vi "Create Custom Device.vi"(0 "Name":string, 5 "AIT 1553 Settings":T2={"Board Serial #"=685, "AppLicense"=FALSE, "License Key"="", "BusEnabledProperties"={"Bus1Enabled"=TRUE, "Bus2Enabled"=FALSE, "Bus3Enabled"=FALSE, "Bus4Enabled"=FALSE}, "Description"="Driver for AIT 1553 Device for VeriStand", "Bus1 Path"=path "", "Bus2 Path"=path "", "Bus3 Path"=path "", "Bus4 Path"=path ""}, 11 "error in (no error)":errorcluster) -> (4 "Custom Device reference":refnum<k24>, 15 "error out":errorcluster)   [LabVIEW 2011]
uses:
  NationalInstruments.VeriStand.SystemDefinitionAPI
  Controls/AIT 1553 Settings.ctl
  System Explorer/Controls/1553 Bus Enabled.ctl
  <vilib>/NI Veristand/Custom Device API/Custom Device Item Ref.ctl
  Controls and Global/Global.vi
  <vilib>/NI Veristand/Custom Device API/Set Item Property (Boolean).vi
  <vilib>/NI Veristand/Custom Device API/Set Item Property (String).vi
  <vilib>/NI Veristand/Custom Device API/Set Item Property (Variant).vi
  <vilib>/NI Veristand/Custom Device API/Custom Device API.lvlib
  AIT 1553 Custom Device.lvlib
panel:
  out "Sim Filenames":path[](array[path])
  out "Bus Nodes":T1[](array[typedef]) format="%.0x"
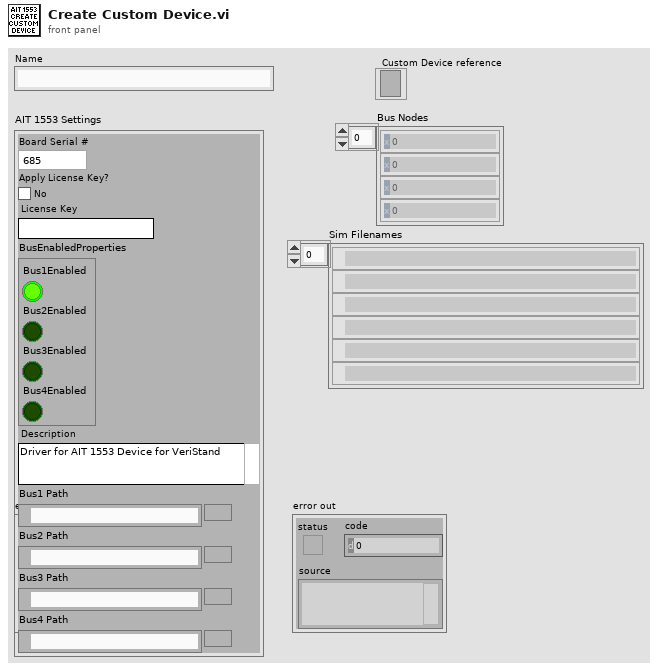
[diagram p1: front panel]
types:
  T1 = typedef "Custom Device API.lvlib/Custom Device Item Ref.ctl" = u64
  T2 = typedef "AIT 1553 Settings.ctl" = cluster{"Board Serial #":u64, "AppLicense":bool, "License Key":string, "BusEnabledProperties":T3, "Description":string, "Bus1 Path":path, "Bus2 Path":path, "Bus3 Path":path, "Bus4 Path":path}
  T3 = typedef "AIT 1553 Custom Device.lvlib/1553 Bus Enabled.ctl" = cluster{"Bus1Enabled":bool, "Bus2Enabled":bool, "Bus3Enabled":bool, "Bus4Enabled":bool}
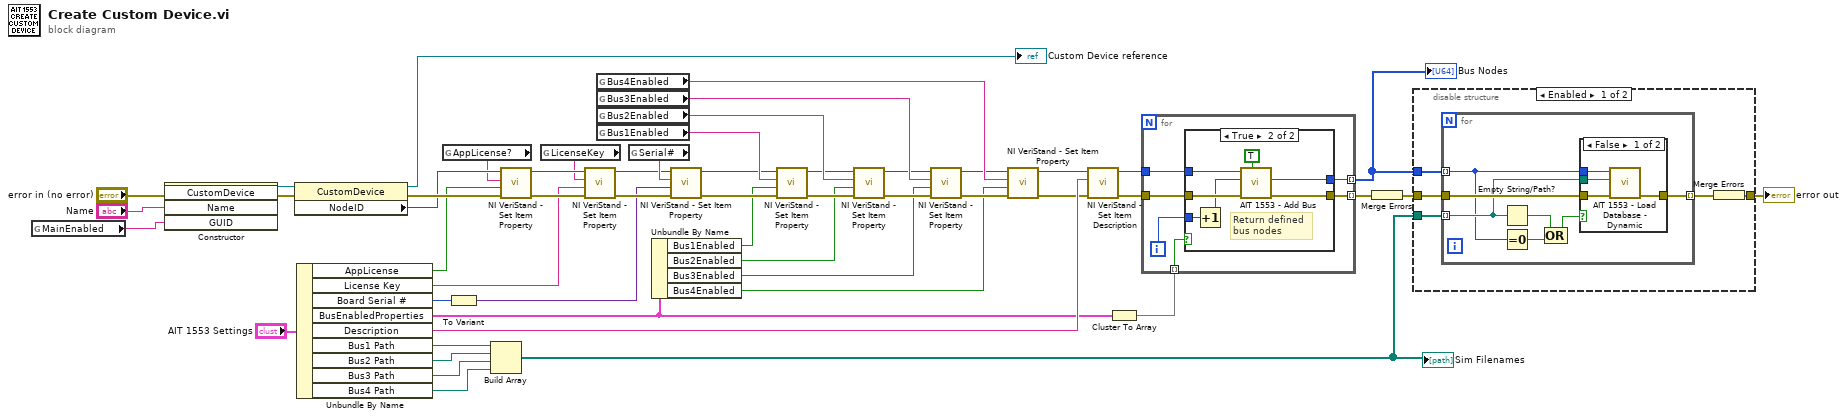
[diagram p0: block diagram]
diagram:
  n1 = global read "Global.vi" "MainEnabled"() -> (w48:string)
  n2 = constructor class="CustomDevice"(error in="error in (no error)", "Name"="Name", "GUID"=w48) -> (reference out=w51:refnum<k24>, error out=w52:errorcluster)  [unwired: 2 in, 3 out]
  n3 = property class="CustomDevice"(reference=w51, error in=w52) -> (reference out=→"Custom Device reference":refnum<k24>, error out=w47:errorcluster, "NodeID"=w44:u64)
  n4 = Unbundle By Name("AIT 1553 Settings") -> ("AppLicense"=w45:bool, "License Key"=w39:string, "Board Serial #"=w36:u64, "BusEnabledProperties"=w14:T3, "Description"=w34:string, "Bus1 Path"=w8:path, "Bus2 Path"=w9:path, "Bus3 Path"=w10:path, "Bus4 Path"=w11:path)
  n5 = global read "Global.vi" "AppLicense?"() -> (w41:string)
  n6 = To Variant(anything=w36) -> (Variant=w35:variant)
  n7 = Build Array(w8, w9, w10, w11) -> (w5:path[])
  "Sim Filenames" <- w5
  n8 = call-poly <vilib>:"NI VeriStand - Set Item Property.vi"("error in (no error)"=w47, "Value"=w45, "Property Name"=w41, "Item Ref in"=w44) -> ("error out"=w42:errorcluster, "Item Ref out"=w43:T1)  [unwired: 5 in, 1 out]
  n9 = global read "Global.vi" "LicenseKey"() -> (w40:string)
  n10 = call-poly <vilib>:"NI VeriStand - Set Item Property.vi"("error in (no error)"=w42, "Value"=w39, "Property Name"=w40, "Item Ref in"=w43) -> ("error out"=w38:errorcluster, "Item Ref out"=w33:T1)  [unwired: 5 in, 1 out]
  n11 = global read "Global.vi" "Bus4Enabled"() -> (w29:string)
  n12 = global read "Global.vi" "Bus3Enabled"() -> (w30:string)
  n13 = global read "Global.vi" "Bus2Enabled"() -> (w31:string)
  n14 = global read "Global.vi" "Bus1Enabled"() -> (w32:string)
  n15 = global read "Global.vi" "Serial#"() -> (w37:string)
  n16 = Unbundle By Name(w14) -> ("Bus1Enabled"=w18:bool, "Bus2Enabled"=w17:bool, "Bus3Enabled"=w16:bool, "Bus4Enabled"=w15:bool)
  n17 = call-poly <vilib>:"NI VeriStand - Set Item Property.vi"("error in (no error)"=w38, "Value"=w35, "Property Name"=w37, "Item Ref in"=w33) -> ("error out"=w27:errorcluster, "Item Ref out"=w28:T1)  [unwired: 5 in, 1 out]
  n18 = call-poly <vilib>:"NI VeriStand - Set Item Property.vi"("error in (no error)"=w27, "Value"=w18, "Property Name"=w32, "Item Ref in"=w28) -> ("error out"=w26:errorcluster, "Item Ref out"=w22:T1)  [unwired: 5 in, 1 out]
  n19 = call-poly <vilib>:"NI VeriStand - Set Item Property.vi"("error in (no error)"=w26, "Value"=w17, "Property Name"=w31, "Item Ref in"=w22) -> ("error out"=w25:errorcluster, "Item Ref out"=w21:T1)  [unwired: 5 in, 1 out]
  n20 = call-poly <vilib>:"NI VeriStand - Set Item Property.vi"("error in (no error)"=w25, "Value"=w16, "Property Name"=w30, "Item Ref in"=w21) -> ("error out"=w24:errorcluster, "Item Ref out"=w20:T1)  [unwired: 5 in, 1 out]
  n21 = call-poly <vilib>:"NI VeriStand - Set Item Property.vi"("error in (no error)"=w24, "Value"=w15, "Property Name"=w29, "Item Ref in"=w20) -> ("error out"=w23:errorcluster, "Item Ref out"=w19:T1)  [unwired: 5 in, 1 out]
  n22 = call <vilib>:"NI VeriStand - Set Item Description.vi"("error in (no error)"=w23, "Description"=w34, "Item Ref in"=w19) -> ("error out"=w7:errorcluster, "Item Ref out"=w6:T1)  [unwired: 7 out]
  n23 = Cluster To Array(cluster=w14) -> (array=w13:bool[])
  n24 = for {
    tunnel: w7 -> [w57]
    tunnel: w6 -> [w58]
    tunnel: w13 -> [w56] mode=indexing
    tunnel: [w54] -> w12 mode=indexing
    tunnel: [w53] -> w1 mode=indexing
    i -> [w55]
    n25 = case shown="True" w56 {
      tunnel: w58 -> [_ w62]
      tunnel: w57 -> [w59 w66]
      tunnel: w55 -> [_ w65]
      tunnel: [w59 w61] -> w54
      tunnel: [_ w60] -> w53
      frame False {
      }
      frame True {
        # "Return defined\nbus nodes"
        n26 = Increment(x=w65) -> (x+1=w64:i32)
        n27 = call "AIT 1553 - Add Bus.vi"("Called From SysDef API (F)"=TRUE, "error in (no error)"=w66, "Bus"=w64, "Node Ptr"=w62) -> ("error out"=w61:errorcluster, "Section Ptr Out"=w60:T1)  [unwired: 6 in]
      }
    }
  }
  "Bus Nodes" <- w1
  n28 = Merge Errors(w12) -> (w2:errorcluster)
  n29 = disable-structure shown="Enabled" {
    disable-tunnel: w5 -> [w71 _]
    disable-tunnel: [w69 w84] -> w4
    disable-tunnel: w2 -> [w68 w84]
    disable-tunnel: w1 -> [w67 _]
    frame Enabled {
      n30 = for {
        tunnel: w68 -> [w78]
        tunnel: w67 -> [w75] mode=indexing
        tunnel: w71 -> [w77] mode=indexing
        tunnel: [w76] -> w70 mode=indexing
        n31 = Empty String/Path?(string/path=w77) -> (empty?=w72:bool)
        n32 = Equal To 0?(x=w75) -> (x = 0?=w74:bool)
        n33 = Compound Arithmetic op=OR(w72, w74) -> (w73:bool)
        n34 = case shown="False" w73 {
          tunnel: w78 -> [w82 w83]
          tunnel: w77 -> [w81 _]
          tunnel: w75 -> [w80 _]
          tunnel: [w79 w83] -> w76
          frame False {
            n35 = call "AIT 1553 - Load Database - Dynamic.vi"("error in (no error)"=w82, "Simulyzer File Path"=w81, "Node Ptr"=w80) -> ("error out"=w79:errorcluster)  [unwired: 8 in]
          }
          frame True {
          }
        }
      }
      n36 = Merge Errors(w70) -> (w69:errorcluster)
    }
    frame Disabled {
    }
  }
  "error out" <- w4
